vi "FlatToRichnidevice_grpc_Session.vi"(5 "OutputClusterType":T1, 11 "InputCluster":T2) -> (3 "OutputCluster":T1)   [LabVIEW 2021, in "NI Switch Client.lvlib"]
uses:
  NI Switch Client.lvlib
  nidevice_grpc_Session_Flat.ctl
  nidevice_grpc_Session.ctl
  nidevice_grpc_Session_session/nidevice_grpc_Session_session.lvclass
  nidevice_grpc_Session_session/nidevice_grpc_Session_session.lvclass/nidevice_grpc_Session_session.ctl
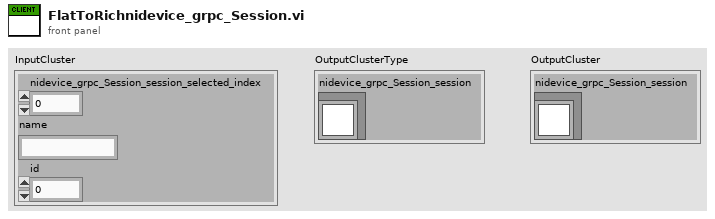
[diagram p1: front panel]
types:
  T1 = typedef "NI Switch Client.lvlib/nidevice_grpc_Session.ctl" = cluster{"nidevice_grpc_Session_session":refnum<class "nidevice_grpc_Session_session.lvclass">}
  T2 = typedef "NI Switch Client.lvlib/nidevice_grpc_Session_Flat.ctl" = cluster{"nidevice_grpc_Session_session_selected_index":i32, "name":string, "id":u32}
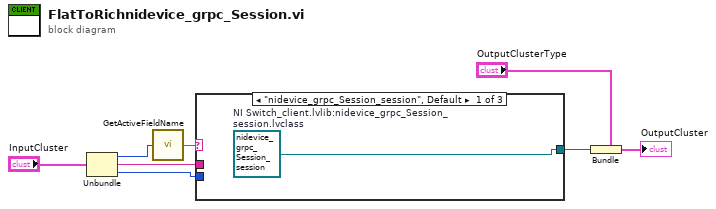
[diagram p0: block diagram]
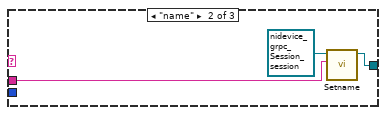
[diagram p2: hidden frame]
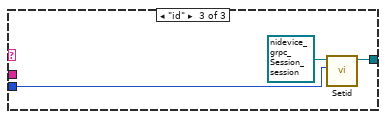
[diagram p3: hidden frame]
diagram:
  n1 = Unbundle "Unbundle"("InputCluster") -> ("nidevice_grpc_Session_session_selected_index"=w5:i32, "name"=w2:string, "id"=w1:u32)
  n2 = call "GetActiveFieldName.vi"("protobuf index"=w5) -> ("oneof field name"=w4:string)
  n3 = case "nidevice_grpc_Session_session" shown="\"nidevice_grpc_Session_session\", Default" w4 {
    tunnel: [w9 w11 w14] -> w3
    tunnel: w2 -> [_ w12 _]
    tunnel: w1 -> [_ _ w15]
    frame "nidevice_grpc_Session_session", Default {
      w9 = refnum<class "nidevice_grpc_Session_session.lvclass"> refnum  # NI Switch_client.lvlib:nidevice_grpc_Session_session.lvclass
    }
    frame "name" {
      n4 = call "Setname.vi"("Set_Val"=w12, "OneOfTemplate in"=refnum<class "nidevice_grpc_Session_session.lvclass"> refnum) -> ("OneOfTemplate out"=w11:refnum<class "nidevice_grpc_Session_session.lvclass">)  [unwired: 8 in, 1 out]
    }
    frame "id" {
      n5 = call "Setid.vi"("Set_Val"=w15, "OneOfTemplate in"=refnum<class "nidevice_grpc_Session_session.lvclass"> refnum) -> ("OneOfTemplate out"=w14:refnum<class "nidevice_grpc_Session_session.lvclass">)  [unwired: 8 in, 1 out]
    }
  }
  n6 = Bundle "Bundle"(cluster="OutputClusterType", "nidevice_grpc_Session_session"=w3) -> (→"OutputCluster":T1)
